vi "USRP Packet Receiver_BER.vi"() -> ()   [LabVIEW 2013]
uses:
  <instrlib>/niUSRP/niUSRP Fetch Rx Data (CDB Cluster).vi
  Global_MessageBits.vi
  <vilib>/addons/Modulation/niDMT.lvlib
panel:
  out "BER":dbl
  out "Packet Array":i32[][](array[numeric])
  out "Actual Rx Parameters":T1 {"Rx Gain [dB]" format="%#.6p"; "Rx\nFrequency [Hz]" format="%#.6p"; "Rx IQ Sampling\nRate [s/sec]" format="%#.6p"}
  in  "Rx Parameters":T1={"Rx IQ Sampling\nRate [s/sec]"=200000.0, "Rx\nFrequency [Hz]"=433920000.0, "Rx Gain [dB]"=0.0, "Rx Antenna"="RX2"} {"Rx Gain [dB]" format="%#.6p"; "Rx\nFrequency [Hz]" format="%#.6p"; "Rx IQ Sampling\nRate [s/sec]" format="%#.6p"}
  out "error out":errorcluster
  in  "USRP IP Address":refnum<k15>
  in  "16-PSK System Parameters":T2={"Samples per Symbol"=8, "symbol map"=[], "Differential PSK"=enum."disable", "PSK type"=0} {"PSK type" items=["normal", "shifted", "offset"]; "symbol map" format="%.3f"}
  in  "8-PSK System Parameters":T2={"Samples per Symbol"=8, "symbol map"=[], "Differential PSK"=enum."disable", "PSK type"=0} {"PSK type" items=["normal", "shifted", "offset"]; "symbol map" format="%.3f"}
  in  "QPSK System Parameters":T2={"Samples per Symbol"=8, "symbol map"=[], "Differential PSK"=enum."disable", "PSK type"=0} {"PSK type" items=["normal", "shifted", "offset"]; "symbol map" format="%.3f"}
  in  "BPSK System Parameters":T2={"Samples per Symbol"=8, "symbol map"=[], "Differential PSK"=enum."disable", "PSK type"=0} {"PSK type" items=["normal", "shifted", "offset"]; "symbol map" format="%.3f"}
  out "Sync Found":bool
  out "Recovered Message":string
  out "Received Signal (Raw)":dbl[](graph)
  out "Constellation Graph":T3(graph)
  in  "filter parameters":T4={"Alpha"=0.5, "Filter Length"=6, "TX Filter"=enum."Root Raised Cos"} caption="Matching Filter Parameters" {"Alpha" format="%.2f"}
  in  "Modulation type":string(combo)="QPSK"
  in  "Acquisition Duration[sec]":dbl=400000.0 format="%#.6p"
  out "Symbol Rate [symbols/sec]":dbl=25000.0 format="%#.6p"
  out "Correct Packets Rx":i16
  in  "Continuous Acquire?":bool
  out "Singal & Noise Power":cluster{"signal_power":dbl, "noise_power":dbl}={"signal_power"=1.4546950663593878e-09, "noise_power"=2.571229598792933e-12}
  out "Cumulative Packets Recovered":i16(graph)
  out "Signal and Noise Power Tracking":cluster{"total_power":dbl, "noise_power":dbl}(graph)={"total_power"=1.4546950663593878e-09, "noise_power"=2.571229598792933e-12}
  in  "PN Sequence Order for Sync":i32=31
  in  "Packet Parameters":T5={"Guard Bits "=30, "Sync Bits"=20, "Message Bits"=128, "Number of Packets \nto Expect"=46}
  in  "synchronization parameters":T6={"expected sync location (symbols)"=-1, "sync sequence"=[], "sync location uncertainty (symbols)"=0, "sync indent (symbols)"=0} {"sync sequence" format="%.2f"}
  in  "stop":bool
  # "Guard\nBand"
  # "Sync\nSeq"
  # "Packet\nNumber"
  # "Pad\nData"
  # "Data"
  # "Packet Receiver"
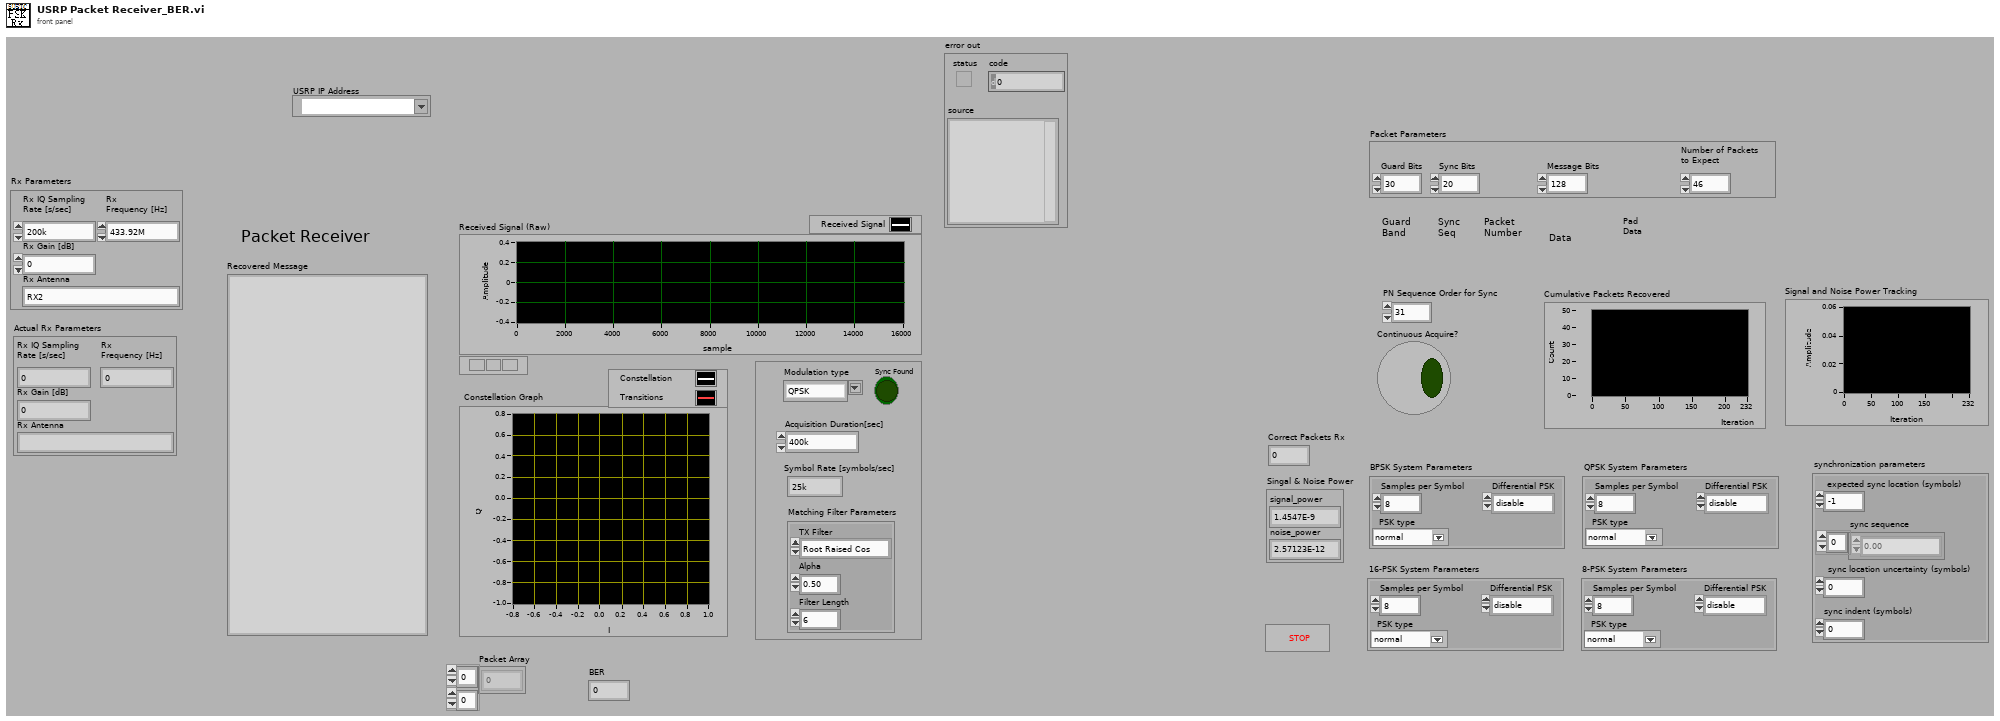
[diagram p1: front panel]
types:
  T1 = cluster{"Rx IQ Sampling\nRate [s/sec]":dbl, "Rx\nFrequency [Hz]":dbl, "Rx Gain [dB]":dbl, "Rx Antenna":string}
  T2 = cluster{"Samples per Symbol":i32, "symbol map":cdb[], "Differential PSK":enum16{"disable", "enable"}, "PSK type":u16}
  T3 = cluster{"Decimated Array":dbl[], "Decimated Array":dbl[]}[]
  T4 = cluster{"Alpha":dbl, "Filter Length":i32, "TX Filter":enum16{"none", "Raised Cosine", "Root Raised Cos", "Gaussian"}}
  T5 = cluster{"Guard Bits ":i32, "Sync Bits":i32, "Message Bits":i32, "Number of Packets \nto Expect":i32}
  T6 = cluster{"expected sync location (symbols)":i32, "sync sequence":cdb[], "sync location uncertainty (symbols)":i32, "sync indent (symbols)":i32}
  T7 = cluster{"Packet Array":i32[][], "IP Array of Pkt Nums Received  ":bool[]}
  T8 = cluster{"bit stream ":i8[][], "Sync Valid?":bool[], "Decoded Pkt Numbers":u32[], "Enable?":bool}
  T9 = cluster{"packet_arr":cdb[][], "Packets Valid?":bool}
  T10 = cluster{"PSK type":u16, "Samples per Symbol":i32, "Differential PSK":enum16{"disable", "enable"}, "M-PSK (4)":i32}
  T11 = cluster{"PSK system parameters":cluster{"samples per symbol (16)":i32, "symbol map":cdb[], "differential PSK":enum16{"disable", "enable"}, "PSK type":u16}, "pulse shaping filter coefficients":dbl[], "matched filter coefficients":dbl[], "synchronization parameters":cluster{"expected sync location (symbols)":i32, "sync sequence":cdb[], "sync location uncertainty (symbols)":i32, "sync indent (symbols)":i32}, "Sync Bits":i8[]}
  T12 = typedef "niAMT.lvlib/Complex Data Waveform.ctl" = cluster{"t0":dbl, "dt":dbl, "Y":cdb[]}
  T13 = cluster{"constellation":dbl[], "oversampled data":dbl[]}[]
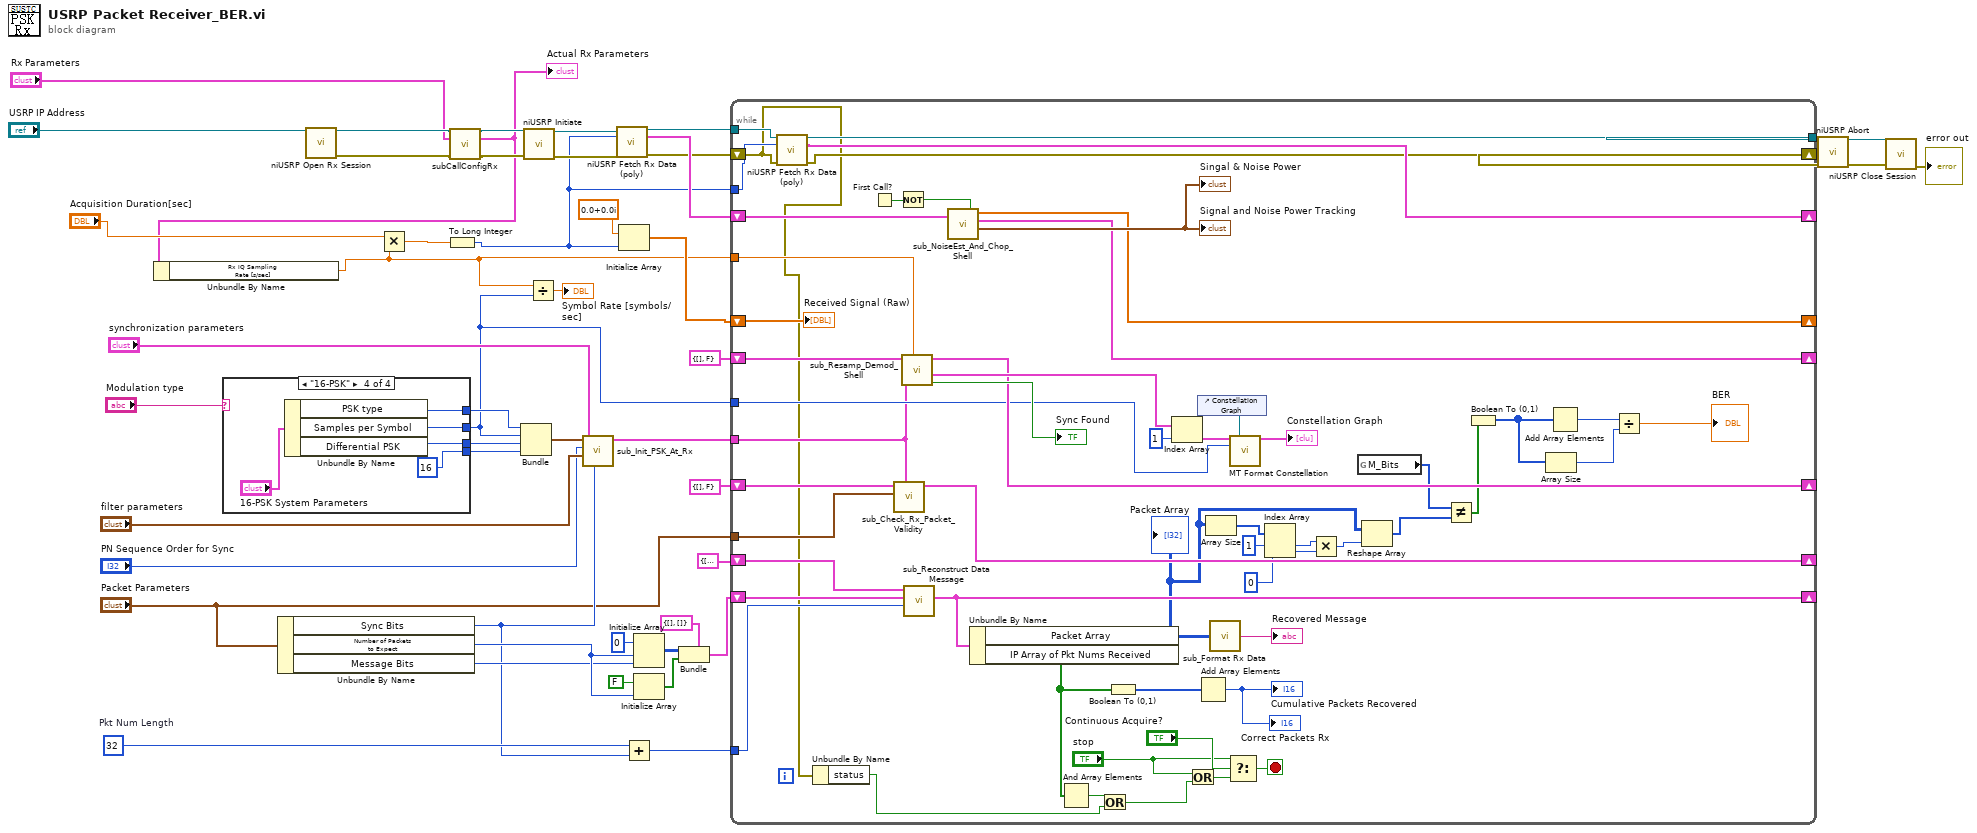
[diagram p0: block diagram]
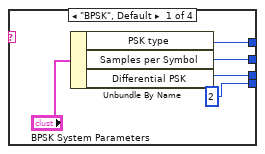
[diagram p2: hidden frame]
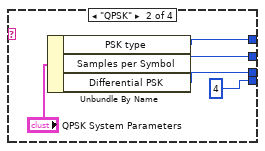
[diagram p3: hidden frame]
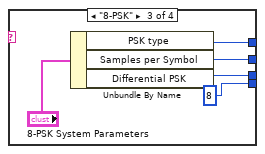
[diagram p4: hidden frame]
diagram:
  w39 = 32  # Pkt Num Length
  n1 = case shown="\"16-PSK\"" "Modulation type" {
    tunnel: [w52 w58 w63 w69] -> w24
    tunnel: [w53 w56 w62 w68] -> w45
    tunnel: [2 ("M-PSK (4)") 4 ("M-PSK (4)") 8 ("M-PSK (4)") 16 ("M-PSK (4)")] -> w44
    tunnel: [w54 w57 w64 w67] -> w46
    frame "BPSK", Default {
      n2 = Unbundle By Name("BPSK System Parameters") -> ("PSK type"=w54:u16, "Samples per Symbol"=w52:i32, "Differential PSK"=w53:enum16{"disable", "enable"})
    }
    frame "QPSK" {
      n3 = Unbundle By Name("QPSK System Parameters") -> ("PSK type"=w57:u16, "Samples per Symbol"=w58:i32, "Differential PSK"=w56:enum16{"disable", "enable"})
    }
    frame "8-PSK" {
      n4 = Unbundle By Name("8-PSK System Parameters") -> ("PSK type"=w64:u16, "Samples per Symbol"=w63:i32, "Differential PSK"=w62:enum16{"disable", "enable"})
    }
    frame "16-PSK" {
      n5 = Unbundle By Name("16-PSK System Parameters") -> ("PSK type"=w67:u16, "Samples per Symbol"=w69:i32, "Differential PSK"=w68:enum16{"disable", "enable"})
    }
  }
  n6 = Unbundle By Name("Packet Parameters") -> ("Sync Bits"=w30:i32, "Number of Packets \nto Expect"=w38:i32, "Message Bits"=w37:i32)
  n7 = call <instrlib>:"niUSRP Open Rx Session.vi"("device names"="USRP IP Address") -> ("session handle out"=w9:refnum<k15>, "error out"=w8:errorcluster)  [unwired: 13 in]
  n8 = call "subCallConfigRx.vi"("session handle"=w9, "Rx Parameters"="Rx Parameters", "error in"=w8) -> ("session handle out"=w7:refnum<k15>, "Actual Rx Parameters"=w2:T1, "error out"=w6:errorcluster)  [unwired: 10 in]
  "Actual Rx Parameters" <- w2
  n9 = Unbundle By Name(w2) -> ("Rx IQ Sampling\nRate [s/sec]"=w3:dbl)
  n10 = Multiply(x="Acquisition Duration[sec]", y=w3) -> (x*y=w4:dbl)
  n11 = To Long Integer(number=w4) -> (32bit integer=w5:i32)
  n12 = Bundle("PSK type"=w46, "Samples per Symbol"=w24, "Differential PSK"=w45, "M-PSK (4)"=w44) -> (w42:T10)  [unwired: 1 in]
  n13 = call <instrlib>:"niUSRP Initiate.vi"("session handle"=w7, "error in (no error)"=w6) -> ("session handle out"=w22:refnum<k15>, "error out"=w21:errorcluster)  [unwired: 12 in]
  n14 = Divide(x=w3, y=w24) -> (x/y=→"Symbol Rate [symbols/sec]":dbl)
  n15 = call "sub_Init_PSK_At_Rx.vi"("Sync Bits"=w30, "synchronization parameters"="synchronization parameters", "filter parameters"="filter parameters", "PN sequence order (9)"="PN Sequence Order for Sync", "PSK Parameters"=w42) -> ("PSK Init Parameters"=w41:T11)  [unwired: 5 in, 1 out]
  n16 = call-poly <instrlib>:"niUSRP Fetch Rx Data (poly).vi"("session handle"=w22, "number of samples"=w5, "error in (no error)"=w21) -> ("session handle out"=w19:refnum<k15>, "data"=w20:cluster{"t0":dbl, "dt":dbl, "Y":cdb[]}, "error out"=w18:errorcluster)  [unwired: 9 in, 1 out]
  n17 = Initialize Array(cdb 0.0+0.0i ("element"), w5) -> (w12:cdb[])
  n18 = Add(x=w39, y=w30) -> (x+y=w47:i32)
  n19 = Initialize Array(0, w38, w37) -> (w32:i32[][])
  n20 = Initialize Array(FALSE, w38) -> (w31:bool[])
  n21 = Bundle(cluster=T7 {"Packet Array"=[], "IP Array of Pkt Nums Received  "=[]} ("Packet Info"), "Packet Array"=w32, "IP Array of Pkt Nums Received"=w31) -> (w27:T7)
  n22 = while {
    tunnel: "Packet Parameters" -> [w125]
    tunnel: w47 -> [w102]
    tunnel: w41 -> [w96]
    tunnel: w24 -> [w97]
    shift-right: [w101] -> _
    shift-left: w27 -> [w103]
    shift-right: [w108] -> _
    shift-left: T9 {"packet_arr"=[], "Packets Valid?"=FALSE} -> [w109]
    shift-right: [w105] -> _
    shift-left: cluster{"bit stream":i8[][], "Enable?":bool} {"bit stream"=[], "Enable?"=FALSE} ("Output Bitstream") -> [w107]
    shift-right: [w95] -> _
    shift-left: T8 {"bit stream "=[], "Sync Valid?"=[], "Decoded Pkt Numbers"=[], "Enable?"=FALSE} ("Output Bit Stream") -> [w104]
    shift-right: [w94] -> _
    shift-left: w20 -> [w106]
    shift-right: [w98] -> _
    shift-left: w12 -> [w99]
    tunnel: w19 -> [w93]
    tunnel: [w92] -> w17
    tunnel: w5 -> [w90]
    shift-right: [w91] -> w16
    shift-left: w18 -> [w86]
    tunnel: w3 -> [w87]
    stop <- w121 stop-if-true
    n23 = call-poly <instrlib>:"niUSRP Fetch Rx Data (poly).vi"("session handle"=w93, "number of samples"=w90, "error in (no error)"=w86) -> ("session handle out"=w92:refnum<k15>, "data"=w94:cluster{"t0":dbl, "dt":dbl, "Y":cdb[]}, "error out"=w91:errorcluster)  [unwired: 9 in, 1 out]
    n24 = Unbundle By Name(w86) -> ("status"=w85:bool)
    n25 = First Call?() -> (First Call?: T/F=w112:bool)
    n26 = call "sub_Check_Rx_Packet_Validity.vi"("PSK Init Parameters"=w96, "Packet Parameters"=w125, "Input Bit Stream"=w107) -> ("Output Bit Stream"=w95:T8)  [unwired: 7 in]
    n27 = Not(x=w112) -> (.not. x?=w111:bool)
    n28 = call "sub_Resamp_Demod_Shell.vi"("Rx IQ Sampling\nRate [s/sec]"=w87, "PSK Init Parameters"=w96, "Input Packets"=w109) -> ("Synch Found?"=→"Sync Found":bool, "recovered complex waveform"=w114:T12[], "Output Bitstream"=w105:cluster{"bit stream":i8[][], "Enable?":bool})  [unwired: 3 in]
    n29 = call "sub_Reconstruct Data Message.vi"("Start Loc of Data"=w102, "Packet Info"=w103, "Input Stream"=w104) -> ("Packet Info out"=w101:T7)  [unwired: 8 in]
    n30 = call "sub_NoiseEst_And_Chop_Shell.vi"("data"=w106, "Enable"=w111) -> ("Singal & Noise Power"=→"Signal and Noise Power Tracking" →"Singal & Noise Power":cluster{"signal_power":dbl, "noise_power":dbl}, "Output Packets"=w108:cluster{"Packets":cdb[][], "Enable?":bool}, "Delay signal (for plotting use only)"=w98:cdb[])  [unwired: 3 in]
    n31 = Unbundle By Name "Unbundle By Name"(w101) -> ("Packet Array"=w80:i32[][], "IP Array of Pkt Nums Received"=w100:bool[])
    "Packet Array" <- w80
    n32 = And Array Elements(Boolean array=w100) -> (logical AND=w88:bool)
    n33 = Or(x=w88, y=w85) -> (x .or. y?=w89:bool)
    n34 = Boolean To (0,1)(Boolean=w100) -> (0, 1=w124:i16[])
    n35 = Index Array(array=w114, index=1) -> (element=w113:T12)
    n36 = Or(x="stop", y=w89) -> (x .or. y?=w122:bool)
    n37 = control-ref of="Constellation Graph"() -> (w116:refnum<vi>)
    n38 = Add Array Elements(numeric array=w124) -> (sum=→"Correct Packets Rx" →"Cumulative Packets Recovered":i16)
    n39 = Array Size(array=w80) -> (size(s)=w81:i32[])
    n40 = call "sub_Format Rx Data.vi"("Output Packet Array"=w80) -> ("Received Message"=→"Recovered Message":string)
    n41 = Select(t="stop", s="Continuous Acquire?", f=w122) -> (s? t:f=w121:bool)
    n42 = call <vilib>:"MT Format Constellation.vi"("waveform"=w113, "constellation reference"=w116, "samples per symbol"=w97) -> ("constellation graph"=→"Constellation Graph":T13)  [unwired: 2 in, 10 out]
    n43 = Index Array(array=w81, index #1=1 ("index"), index #2=0 ("index")) -> (element #1=w78:i32, element #2=w77:i32)
    n44 = Multiply(x=w78, y=w77) -> (x*y=w79:i32)
    n45 = global read "Global_MessageBits.vi" "M_Bits"() -> (w71:i8[])
    n46 = Reshape Array(w80, w79) -> (w70:i32[])
    n47 = Not Equal?(x=w71, y=w70) -> (x != y?=w76:bool[])
    n48 = Boolean To (0,1)(Boolean=w76) -> (0, 1=w73:i16[])
    n49 = Array Size(array=w73) -> (size(s)=w72:i32)
    n50 = Add Array Elements(numeric array=w73) -> (sum=w75:i16)
    n51 = Divide(x=w75, y=w72) -> (x/y=→"BER":dbl)
    "Received Signal (Raw)" <- w99
  }
  n52 = call <instrlib>:"niUSRP Abort.vi"("session handle"=w17, "error in (no error)"=w16) -> ("session handle out"=w15:refnum<k15>, "error out"=w14:errorcluster)  [unwired: 12 in]
  n53 = call <instrlib>:"niUSRP Close Session.vi"("session handle"=w15, "error in (no error)"=w14) -> ("error out"=→"error out":errorcluster)  [unwired: 13 in]
